vi "convert output indicies to typedef data.vi"(11 "Input Mapping Info":T1) -> (3 "Outputs to system":T2)   [LabVIEW 2013, in "fixed channel tag bus module.lvclass"]
uses:
  fixed channel tag bus module.lvclass
  outputs.ctl
  Channel Run Time Mapping Info.ctl
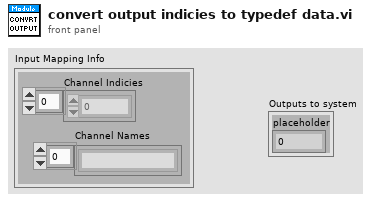
[diagram p1: front panel]
types:
  T1 = typedef "fixed channel tag bus module.lvclass/Channel Run Time Mapping Info.ctl" = cluster{"Channel Indicies":i32[], "Channel Names":string[]}
  T2 = typedef "fixed channel tag bus module.lvclass/outputs.ctl" = cluster{"placeholder":i32}
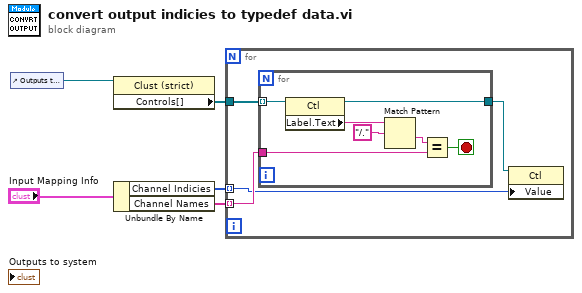
[diagram p0: block diagram]
diagram:
  n1 = control-ref of="Outputs to system"() -> (w2:refnum<vi>)
  n2 = property class="Clust (strict)"(reference=w2) -> ("Controls[]"=w5:refnum<vi>[])  [unwired: 1 in, 2 out]
  n3 = Unbundle By Name("Input Mapping Info") -> ("Channel Indicies"=w3:i32[], "Channel Names"=w4:string[])
  n4 = for {
    tunnel: w5 -> [w9]
    tunnel: w4 -> [w8] mode=indexing
    tunnel: w3 -> [w6] mode=indexing
    n5 = for {
      tunnel: w9 -> [w16] mode=indexing
      tunnel: w8 -> [w12]
      tunnel: [w10] -> w7
      stop <- w11 stop-if-true
      n6 = property class="Ctl"(reference=w16) -> (reference out=w10:refnum<vi>, "Label.Text"=w15:string)  [unwired: 1 in, 1 out]
      n7 = Match Pattern(string=w15, regular expression="/.") -> (after substring=w13:string)  [unwired: 1 in, 3 out]
      n8 = Equal?(x=w13, y=w12) -> (x = y?=w11:bool)
    }
    n9 = property class="Ctl"(reference=w7, "Value"=w6) -> ()  [unwired: 1 in, 2 out]
  }
